vi "CLSUIP_StripExtension.vi"(1 "string":string) -> (0 "string without extension":string)   [LabVIEW 2021, in "MemberVICreation.lvlib" / "VIRetooler.lvclass"]
uses:
  <resource>/Framework/Providers/LVClassLibrary/NewAccessors/VIRetooler/VIRetooler.lvclass
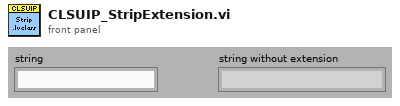
[diagram p1: front panel]
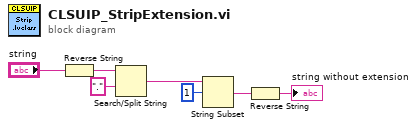
[diagram p0: block diagram]
diagram:
  n1 = Reverse String(1:"string") -> (0:w5:string)
  n2 = Search/Split String(string=w5, search string/char (-)=".") -> (match + rest of string=w3:string)  [unwired: 3 out]
  n3 = String Subset(string=w3, offset (0)=1) -> (substring=w2:string)  [unwired: 1 out]
  n4 = Reverse String(1:w2) -> (0:→"string without extension":string)
